vi "Locate STX.vi"(11 "Array":i32[](array[numeric])) -> ()   [LabVIEW 2016]
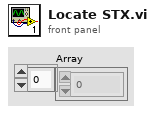
[diagram p1: front panel]
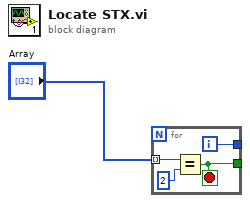
[diagram p0: block diagram]
diagram:
  n1 = for {
    tunnel: "Array" -> [w5] mode=indexing
    tunnel: [w3] -> _
    tunnel: [w2] -> _
    i -> [w2]
    stop <- w3 stop-if-true
    n2 = Equal?(x=w5, y=u8 2) -> (x = y?=w3:bool)
  }
